vi "BRig_dataBlock_nTrial_PostR.vi"() -> (2 "output_nTrial_PostR":i32)   [LabVIEW 2014]
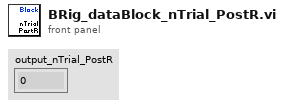
[diagram p1: front panel]
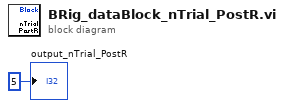
[diagram p0: block diagram]
diagram:
  "output_nTrial_PostR" <- 5 ("output_iBlock")
